vi "Get Operation.vi"(8 "error in (no error)":errorcluster) -> (0 "error out":errorcluster, 1 "Data":variant, 2 "Operation":string, 3 "Section":string)   [LabVIEW 2014]
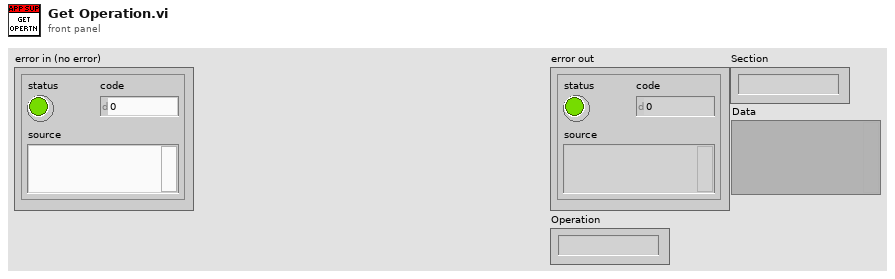
[diagram p1: front panel]
types:
  T1 = typedef "Data Queue.ctl" = cluster{"Command":string, "Data":variant}
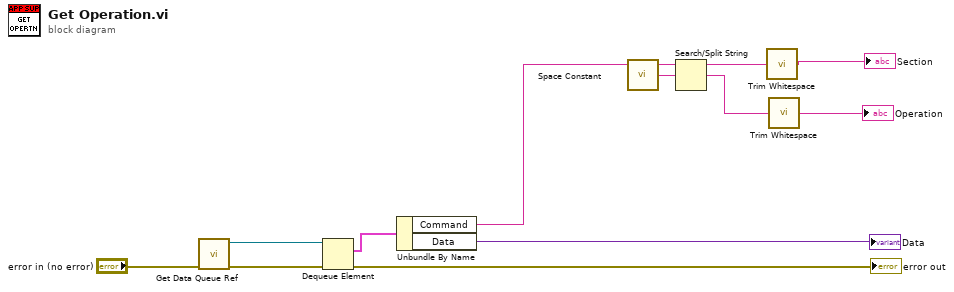
[diagram p0: block diagram]
diagram:
  n1 = call "Get Data Queue Ref.vi"("error in (no error)"="error in (no error)") -> ("error out"=w10:errorcluster, "Ground Station Operations Queue Ref"=w11:refnum<queue>)  [unwired: 9 in]
  n2 = Dequeue Element(queue=w11, error in (no error)=w10) -> (element=w8:T1, error out=→"error out":errorcluster)  [unwired: 1 in, 2 out]
  n3 = Unbundle By Name(w8) -> ("Command"=w6:string, "Data"=→"Data":variant)
  n4 = call <vilib>:"Space Constant.vi"() -> ("String"=w3:string)
  n5 = Search/Split String(string=w6, search string/char (-)=w3) -> (substring before match=w5:string, match + rest of string=w4:string)  [unwired: 1 in, 1 out]
  n6 = call <vilib>:"Trim Whitespace.vi"("string"=w5) -> ("trimmed string"=→"Section":string)  [unwired: 1 in]
  n7 = call <vilib>:"Trim Whitespace.vi"("string"=w4) -> ("trimmed string"=→"Operation":string)  [unwired: 1 in]
